vi "Update Recent Config File Paths.vi"(8 "error in":errorcluster, 11 "configuration files page data":T1 {"custom device ref" format="%.0x"}) -> (0 "error out":errorcluster, 3 "configuration files page data out":T1 {"custom device ref" format="%.0x"})   [LabVIEW 2020, in "Ballard ARINC 429 System Explorer.lvlib" / "Implementation.lvlib"]
uses:
  Implementation.lvlib
  Types/Configuration Files Page Data.ctl
  Types/Path Control.ctl
  Types/Browse Button.ctl
  <vilib>/NI VeriStand/Custom Device API/Custom Device Item Ref.ctl
  <vilib>/NI VeriStand/Custom Device API/Custom Device API.lvlib
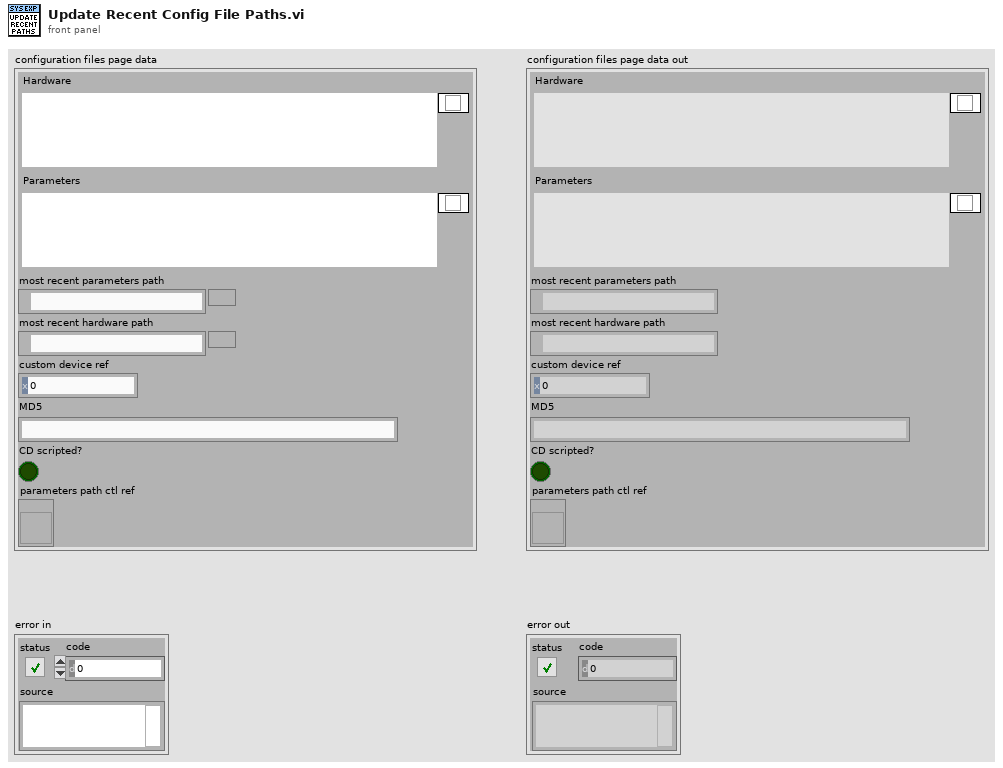
[diagram p1: front panel]
types:
  T1 = typedef "Ballard ARINC 429 System Explorer.lvlib/Implementation.lvlib/Configuration Files Page Data.ctl" = cluster{"Hardware":T2, "Parameters":T2, "most recent parameters path":path, "most recent hardware path":path, "custom device ref":T4, "MD5":string, "CD scripted?":bool, "parameters path ctl ref":refnum<vi>}
  T2 = typedef "Ballard ARINC 429 System Explorer.lvlib/Implementation.lvlib/Path Control.ctl" = cluster{"file path":path, "Browse":T3}
  T3 = typedef "Ballard ARINC 429 System Explorer.lvlib/Implementation.lvlib/Browse Button.ctl" = bool
  T4 = typedef "Custom Device API.lvlib/Custom Device Item Ref.ctl" = u64
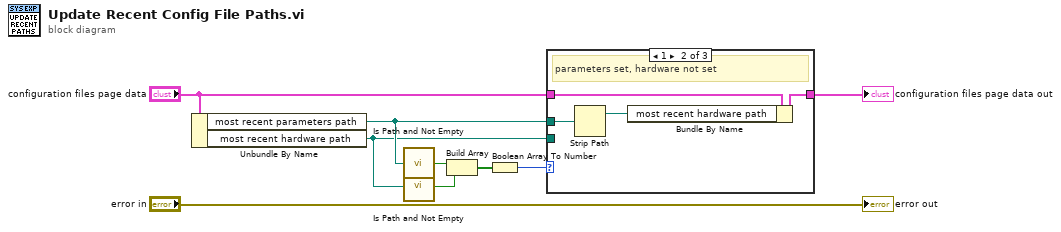
[diagram p0: block diagram]
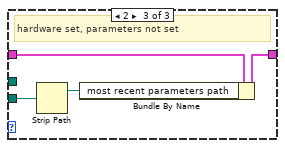
[diagram p3: hidden frame]
diagram:
  n1 = Unbundle By Name("configuration files page data") -> ("most recent parameters path"=w5:path, "most recent hardware path"=w4:path)
  n2 = call <vilib>:"Is Path and Not Empty.vi"("path"=w5) -> ("Is Path and Not Empty?"=w9:bool)  [unwired: 4 in]
  n3 = call <vilib>:"Is Path and Not Empty.vi"("path"=w4) -> ("Is Path and Not Empty?"=w8:bool)  [unwired: 4 in]
  n4 = Build Array(w9, w8) -> (w7:bool[])
  n5 = Boolean Array To Number(Boolean array=w7) -> (number=w6:u32)
  n6 = case shown="1" w6 {
    tunnel: w5 -> [_ w13 _]
    tunnel: w4 -> [_ _ w15]
    tunnel: "configuration files page data" -> [w10 w14 w18]
    tunnel: [w10 w11 w16] -> w2
    frame Default {
      # "Neither is set or both are set"
    }
    frame 1 {
      # "parameters set, hardware not set"
      n7 = Strip Path(path=w13) -> (stripped path=w12:path)  [unwired: 1 out]
      n8 = Bundle By Name(cluster=w14, "most recent hardware path"=w12) -> (w11:T1)
    }
    frame 2 {
      # "hardware set, parameters not set"
      n9 = Strip Path(path=w15) -> (stripped path=w17:path)  [unwired: 1 out]
      n10 = Bundle By Name(cluster=w18, "most recent parameters path"=w17) -> (w16:T1)
    }
  }
  "configuration files page data out" <- w2
  "error out" <- "error in"
